vi "test3.vi"() -> ()   [LabVIEW 2023]
panel:
  out "value":T1
  in  "Config file path":path
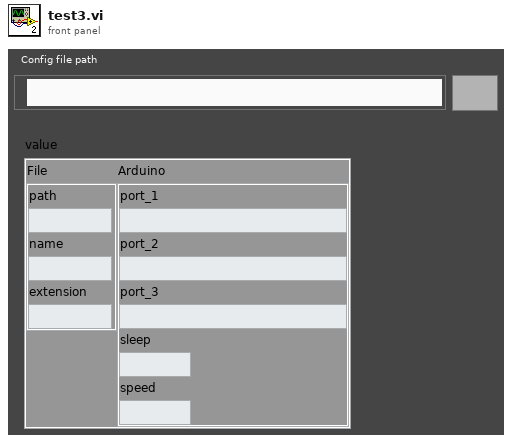
[diagram p1: front panel]
types:
  T1 = cluster{"File":cluster{"path":string, "name":string, "extension":string}, "Arduino":cluster{"port_1":string, "port_2":string, "port_3":string, "sleep":string, "speed":string}}
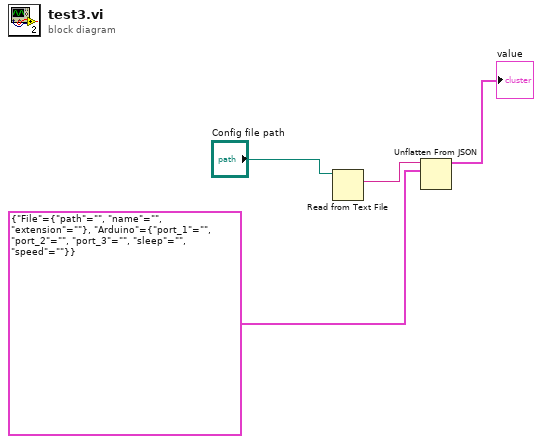
[diagram p0: block diagram]
diagram:
  n1 = Read from Text File(file (use dialog)="Config file path") -> (text=w4:string)  [unwired: 3 in, 3 out]
  n2 = Unflatten From JSON(JSON string=w4, type and defaults=T1 {"File"={"path"="", "name"="", "extension"=""}, "Arduino"={"port_1"="", "port_2"="", "port_3"="", "sleep"="", "speed"=""}}) -> (value=→"value":T1)  [unwired: 5 in, 1 out]
